vi "parseQuickKey_V0.vi"(8 "error in (no error)":errorcluster, 11 "Hexadecimal String":string) -> (0 "error out":errorcluster, 1 "BitCount":i32, 2 "ByteCount":i32, 3 "BinaryArray":string[](array[string]))   [LabVIEW 2018]
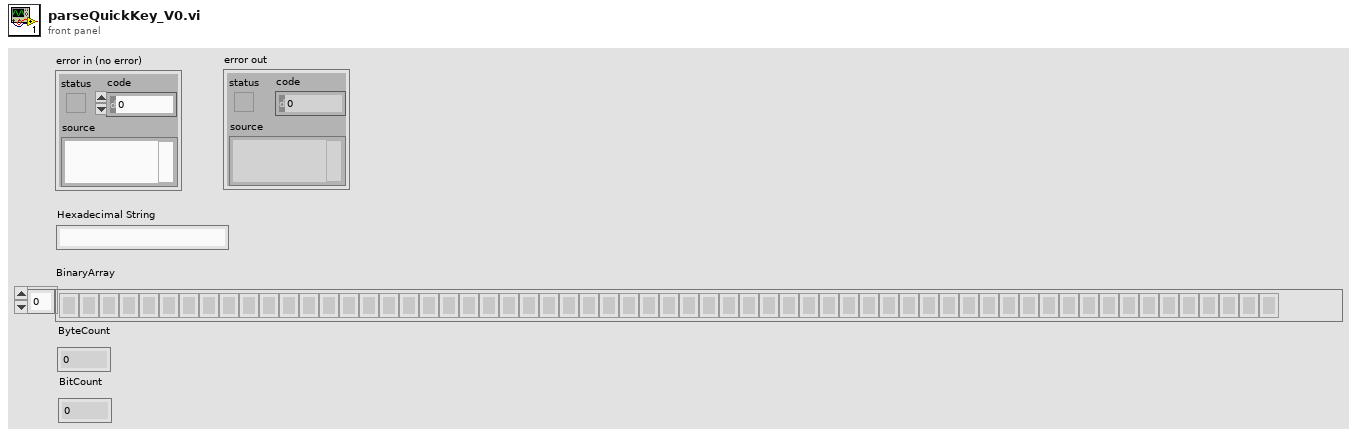
[diagram p1: front panel]
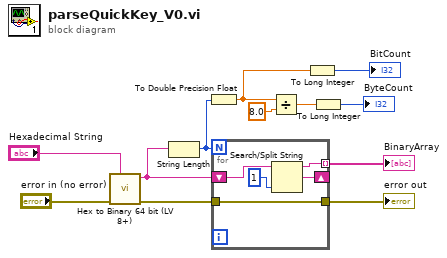
[diagram p0: block diagram]
diagram:
  n1 = call "Hex to Binary 64 bit (LV 8+).vi"("error in (no error)"="error in (no error)", "Hexadecimal String"="Hexadecimal String") -> ("error out"=w5:errorcluster, "Binary String"=w8:string)  [unwired: 5 in, 1 out]
  n2 = String Length(string=w8) -> (length=w12:i32)
  n3 = To Double Precision Float(number=w12) -> (double precision float=w11:dbl)
  n4 = for {
    N: w12 -> [_]
    shift-right: [w17] -> _
    shift-left: w8 -> [w16]
    tunnel: [w15] -> w7 mode=indexing
    tunnel: [w13] -> w4
    tunnel: w5 -> [w13]
    n5 = Search/Split String(string=w16, offset (0)=1) -> (substring before match=w15:string, match + rest of string=w17:string)  [unwired: 1 in, 1 out]
  }
  "BinaryArray" <- w7
  "error out" <- w4
  n6 = Divide(x=w11, y=8.0) -> (x/y=w9:dbl)
  n7 = To Long Integer(number=w11) -> (32bit integer=→"BitCount":i32)
  n8 = To Long Integer(number=w9) -> (32bit integer=→"ByteCount":i32)
